vi "main_MDIsystem.vi"() -> ()   [LabVIEW 2009]
uses:
  FG states.ctl
  MDI_global.vi
  <vilib>/Utility/miscctls.llb/LVBoundsTypeDef.ctl
  <vilib>/Utility/miscctls.llb/LVRectTypeDef.ctl
panel:
  in  "Close app":bool
  in  "window list":u16(ring)
  in  "Remove child window":bool
  in  "Create Child window":bool
  in  "-dummy":bool
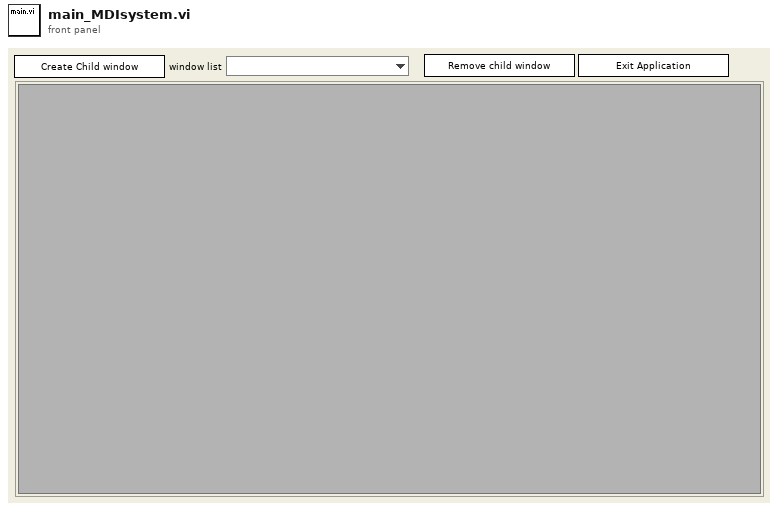
[diagram p1: front panel]
types:
  T1 = typedef "FG states.ctl" = enum16{"init", "add", "replace", "remove", "read"}
  T2 = typedef "LVBoundsTypeDef.ctl" = cluster{"Width":u32, "Height":u32}
  T3 = typedef "LVRectTypeDef.ctl" = cluster{"Left":i16, "Top":i16, "Right":i16, "Bottom":i16}
  T4 = enum32{"Invalid", "Standard", "Closed", "Hidden", "Minimized", "Maximized"}
  T5 = typedef "LVPositionTypeDef.ctl" = cluster{"Left":i32, "Top":i32}
  T6 = typedef "child window props.ctl" = cluster{"WindowTitle":string, "hWnd":u32, "VI Refnum":refnum<vi>}
  T7 = cluster{"Vi tiltle":string, "hWnd":u32, "vi reference out (dup)":refnum<vi>}
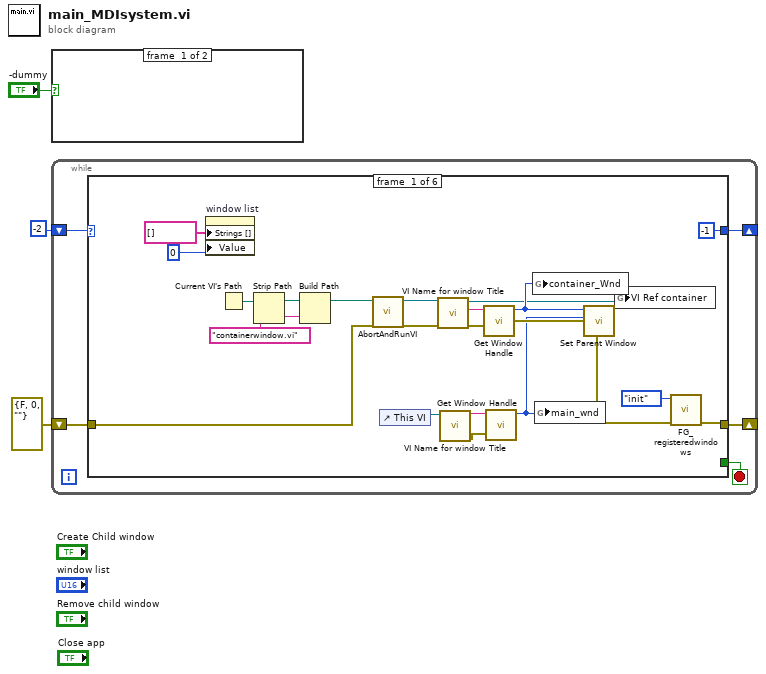
[diagram p0: block diagram]
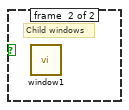
[diagram p2: hidden frame]
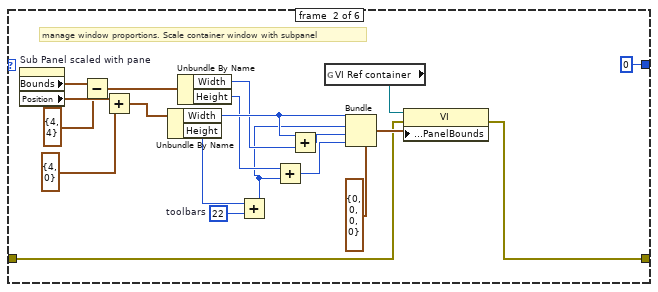
[diagram p3: hidden frame]
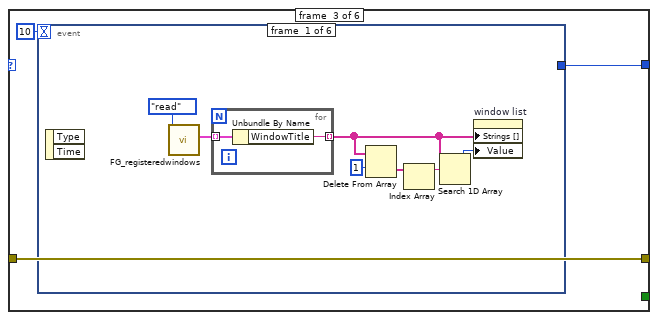
[diagram p4: hidden frame]
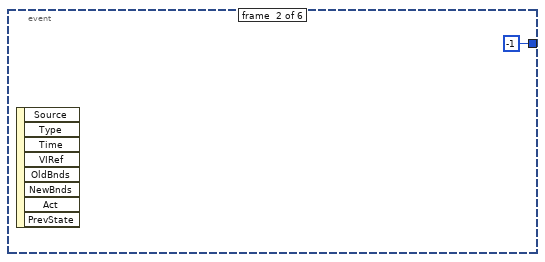
[diagram p5: hidden frame]
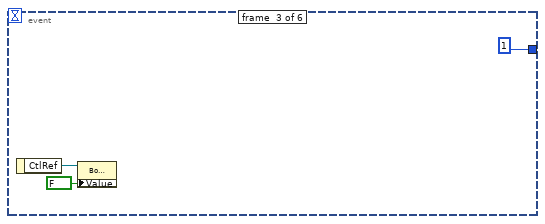
[diagram p6: hidden frame]
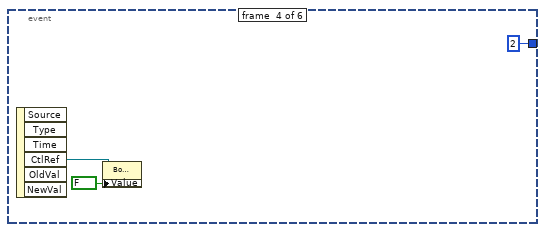
[diagram p7: hidden frame]
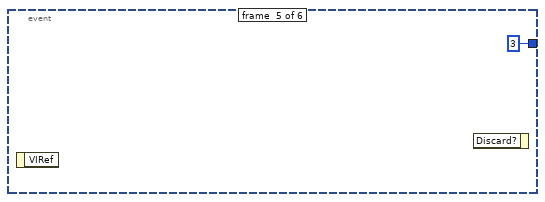
[diagram p8: hidden frame]
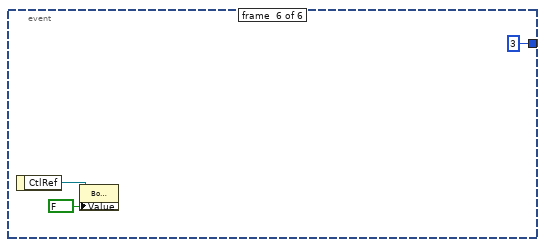
[diagram p9: hidden frame]
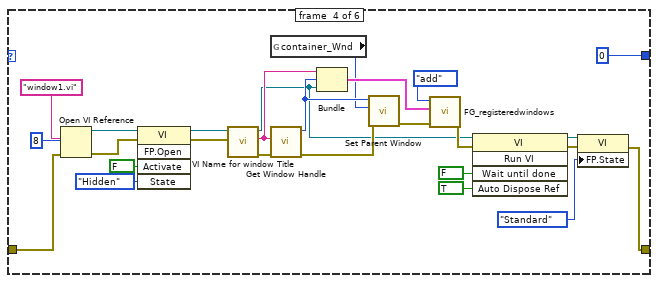
[diagram p10: hidden frame]
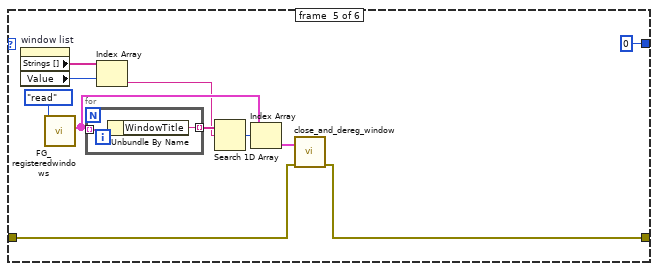
[diagram p11: hidden frame]
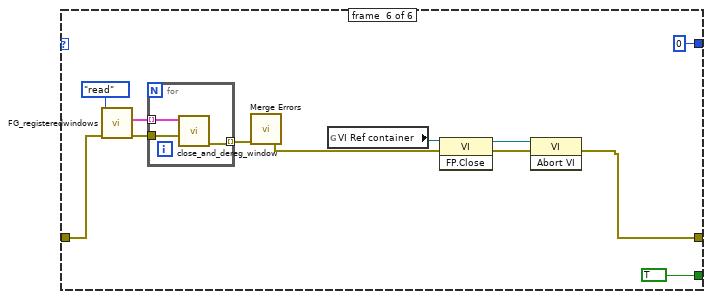
[diagram p12: hidden frame]
diagram:
  n1 = case shown="True" "-dummy" {
    frame #0 {
    }
    frame #1 {
      # "Child windows"
      n2 = call "window1.vi"() -> ()  [unwired: 1 out]
    }
  }
  n3 = while {
    shift-right: [w5] -> _
    shift-left: -2 -> [w8]
    shift-right: [w6] -> _
    shift-left: errorcluster {"status"=FALSE, "code"=0, "source"=""} ("error out") -> [w7]
    stop <- w4 stop-if-true
    n4 = case shown="1" w8 {
      tunnel: w7 -> [w14 w41 w51 w91 w109 w116]
      tunnel: [w25 w40 w51 w74 w102 w112] -> w6
      tunnel: [-1 0 w52 0 0 0] -> w5
      tunnel: [_ _ _ _ _ TRUE] -> w4
      frame #0 {
        n5 = property on="window list" class="Ring (strict)"("Strings []"=string[] [], "Value"=0) -> ()  [unwired: 2 in, 2 out]
        n6 = Current VI's Path() -> (path=w27:path)
        n7 = Strip Path(path=w27) -> (stripped path=w26:path)  [unwired: 1 out]
        n8 = Build Path(base path=w26, name or relative path="containerwindow.vi" ("vi path")) -> (appended path=w13:path)
        n9 = call "AbortAndRunVI.vi"("error out"=w14, "appended path"=w13) -> ("error out 4"=w11:errorcluster, "vi reference 4"=w12:refnum<vi>)  [unwired: 8 out]
        n10 = control-ref of="This VI"() -> (w24:refnum<vi>)
        n11 = call "VI Name for window Title.vi"("error in"=w11, "vi reference"=w12) -> ("error out"=w16:errorcluster, "Vi tiltle"=w21:string, "vi reference out (dup)"=w17:refnum<vi>)  [unwired: 7 out]
        n12 = call "VI Name for window Title.vi"("vi reference"=w24) -> ("error out"=w15:errorcluster, "Vi tiltle"=w23:string)  [unwired: 1 in, 8 out]
        n13 = call "Get Window Handle.vi"("error in (no error)"=w16, "window name (\"\")"=w21) -> ("error out"=w20:errorcluster, "hWnd"=w18:u32)  [unwired: 1 in, 3 out]
        n14 = call "Get Window Handle.vi"("error in (no error)"=w15, "window name (\"\")"=w23) -> ("hWnd"=w19:u32)  [unwired: 1 in, 4 out]
        n15 = global write "MDI_global.vi" "container_Wnd"(w18) -> ()
        n16 = global write "MDI_global.vi" "main_wnd"(w19) -> ()
        n17 = call "Set Parent Window.vi"("new parent"=w19, "child"=w18) -> ()  [unwired: 2 in, 8 out]
        n18 = global write "MDI_global.vi" "VI Ref container"(w17) -> ()
        n19 = call "FG_registeredwindows.vi"("error in (no error)"=w20, "action"=FG_states."init") -> ("error out"=w25:errorcluster)  [unwired: 1 in, 8 out]
      }
      frame #1 {
        w38 = u32 22  # toolbars
        # "manage window proportions. Scale container window with subpanel"
        n20 = property on="Sub Panel scaled with pane" class="SubPnl"() -> ("Bounds"=w35:T2, "Position"=w33:T5)  [unwired: 2 in, 2 out]
        n21 = Subtract(x=w35, y=T2 {"Width"=4, "Height"=4}) -> (x-y=w34:T2)
        n22 = Add(x=w33, y=T2 {"Width"=4, "Height"=0}) -> (x+y=w32:T2)
        n23 = Unbundle By Name(w32) -> ("Width"=w48:u32, "Height"=w37:u32)
        n24 = Unbundle By Name(w34) -> ("Width"=w47:u32, "Height"=w46:u32)
        n25 = Add(x=w37, y=w38) -> (x+y=w36:u32)
        n26 = Add(x=w46, y=w36) -> (x+y=w39:u32)
        n27 = Add(x=w48, y=w47) -> (x+y=w45:u32)
        n28 = global read "MDI_global.vi" "VI Ref container"() -> (w43:refnum<vi>)
        n29 = Bundle(cluster=T3 {"Left"=0, "Top"=0, "Right"=0, "Bottom"=0} ("Front Panel Window:Panel Bounds"), "Left"=w48, "Top"=w36, "Right"=w45, "Bottom"=w39) -> (w44:T3)
        n30 = property class="VI"(reference=w43, error in=w41, "Front Panel.PanelBounds"=w44) -> (error out=w40:errorcluster)  [unwired: 1 out]
      }
      frame #2 {
        n31 = event shown="[3] \"Remove child window\": Value Change" {
          selector: _ -> [_ _ _ _ _ _]
          dyn-events: _ -> [_ _ _ _ _ _]
          timeout: 10 -> [_ _ _ _ _ _]
          tunnel: [_ -1 1 2 3 3] -> w52
          event #0 {
            n32 = event-data() -> ()  [unwired: 3 out]
            n33 = call "FG_registeredwindows.vi"("action"=FG_states."read") -> ("windows"=w58:T6[])  [unwired: 2 in, 8 out]
            n34 = for {
              tunnel: w58 -> [w61] mode=indexing
              tunnel: [w60] -> w55 mode=indexing
              n35 = Unbundle By Name(w61) -> ("WindowTitle"=w60:string)
            }
            n36 = Delete From Array(array=w55, length=1) -> (deleted portion=w56:string[])  [unwired: 1 in, 1 out]
            n37 = Index Array(array=w56) -> (element=w54:string)  [unwired: 1 in]
            n38 = Search 1D Array(1D array=w55, element=w54) -> (index of element=w53:i32)  [unwired: 1 in]
            n39 = property on="window list" class="Ring (strict)"("Strings []"=w55, "Value"=w53) -> ()  [unwired: 2 in, 2 out]
          }
          event #1 {
            n40 = event-data() -> ()  [unwired: 9 out]
          }
          event #2 {
            n41 = event-data() -> ("CtlRef"=w64:refnum<vi>)  [unwired: 1 out]
            n42 = property class="Bool (strict)"(reference=w64, "Value"=FALSE) -> ()  [unwired: 1 in, 2 out]
          }
          event #3 {
            n43 = event-data() -> ("CtlRef"=w66:refnum<vi>)  [unwired: 6 out]
            n44 = property class="Bool (strict)"(reference=w66, "Value"=FALSE) -> ()  [unwired: 1 in, 2 out]
          }
          event #4 {
            n45 = event-data() -> ()  [unwired: 2 out]
            n46 = event-data() -> ()  [unwired: 1 in, 2 out]
          }
          event #5 {
            n47 = event-data() -> ("CtlRef"=w70:refnum<vi>)  [unwired: 1 out]
            n48 = property class="Bool (strict)"(reference=w70, "Value"=FALSE) -> ()  [unwired: 1 in, 2 out]
          }
        }
      }
      frame #3 {
        n49 = Open VI Reference(vi path="window1.vi", options=8, error in (no error)=w91) -> (vi reference=w86:refnum<vi>, error out=w85:errorcluster)  [unwired: 3 out]
        n50 = invoke class="VI" method="FP.Open"(reference=w86, error in=w85, "Activate"=FALSE ("Activate?"), "State"=T4."Hidden") -> (reference out=w84:refnum<vi>, error out=w83:errorcluster)  [unwired: 1 in, 3 out]
        n51 = call "VI Name for window Title.vi"("error in"=w83, "vi reference"=w84) -> ("error out"=w90:errorcluster, "Vi tiltle"=w88:string, "vi reference out (dup)"=w79:refnum<vi>)  [unwired: 7 out]
        n52 = global read "MDI_global.vi" "container_Wnd"() -> (w87:u32)
        n53 = call "Get Window Handle.vi"("error in (no error)"=w90, "window name (\"\")"=w88) -> ("error out"=w89:errorcluster, "hWnd"=w96:u32)  [unwired: 1 in, 3 out]
        n54 = Bundle("Vi tiltle"=w88, "hWnd"=w96, "vi reference out (dup)"=w79) -> (w94:T7)  [unwired: 1 out]
        n55 = call "Set Parent Window.vi"("error in (no error)"=w89, "new parent"=w87, "child"=w96) -> ("error out"=w93:errorcluster)  [unwired: 1 in, 7 out]
        n56 = call "FG_registeredwindows.vi"("error in (no error)"=w93, "window"=w94, "action"=FG_states."add") -> ("error out"=w82:errorcluster)  [unwired: 8 out]
        n57 = invoke class="VI" method="Run VI"(reference=w79, error in=w82, "Wait until done"=FALSE ("Wait Until Done"), "Auto Dispose Ref"=TRUE ("Auto Dispose Reference")) -> (reference out=w75:refnum<vi>, error out=w76:errorcluster)  [unwired: 1 in, 3 out]
        n58 = property class="VI"(reference=w75, error in=w76, "FP.State"=T4."Standard" ("Front Panel Window:State")) -> (error out=w74:errorcluster)  [unwired: 1 out]
      }
      frame #4 {
        n59 = property on="window list" class="Ring (strict)"() -> ("Strings []"=w101:string[], "Value"=w100:u16)  [unwired: 2 in, 2 out]
        n60 = call "FG_registeredwindows.vi"("action"=FG_states."read") -> ("windows"=w105:T6[])  [unwired: 2 in, 8 out]
        n61 = for {
          tunnel: w105 -> [w111] mode=indexing
          tunnel: [w110] -> w106 mode=indexing
          n62 = Unbundle By Name(w111) -> ("WindowTitle"=w110:string)
        }
        n63 = Index Array(array=w101, index=w100) -> (element=w99:string)
        n64 = Search 1D Array(1D array=w106, element=w99) -> (index of element=w104:i32)  [unwired: 1 out]
        n65 = Index Array(array=w105, index=w104) -> (element=w103:T6)
        n66 = call "close_and_dereg_window.vi"("error in"=w109, "window"=w103) -> ("error out"=w102:errorcluster)  [unwired: 8 out]
      }
      frame #5 {
        n67 = call "FG_registeredwindows.vi"("error in (no error)"=w116, "action"=FG_states."read") -> ("error out"=w118:errorcluster, "windows"=w119:T6[])  [unwired: 1 in, 7 out]
        n68 = for {
          tunnel: w119 -> [w126] mode=indexing
          tunnel: w118 -> [w125]
          tunnel: [w124] -> w117 mode=indexing
          n69 = call "close_and_dereg_window.vi"("error in"=w125, "window"=w126) -> ("error out"=w124:errorcluster)  [unwired: 8 out]
        }
        n70 = call <vilib>:"Merge Errors.vi"("error array in"=w117) -> ("error out"=w115:errorcluster)  [unwired: 3 in, 3 out]
        n71 = global read "MDI_global.vi" "VI Ref container"() -> (w121:refnum<vi>)
        n72 = invoke class="VI" method="FP.Close"(reference=w121, error in=w115) -> (reference out=w114:refnum<vi>, error out=w113:errorcluster)  [unwired: 1 in, 1 out]
        n73 = invoke class="VI" method="Abort VI"(reference=w114, error in=w113) -> (error out=w112:errorcluster)  [unwired: 1 in, 2 out]
      }
    }
  }
